vi "Open.vi"(8 "error in (no error)":errorcluster, 11 "Ini-File in":refnum<class "Ini-File.lvclass">) -> (0 "error out":errorcluster, 3 "Ini-File out":refnum<class "Ini-File.lvclass">)   [LabVIEW 2016, in "Configuration.lvlib" / "Ini-File.lvclass"]
doc: "Open connection to ini-file."
uses:
  Ini-File.lvclass
  Ini-File.lvclass/Ini-File.ctl
  <vilib>/Utility/config.llb/NI_LVConfig.lvlib
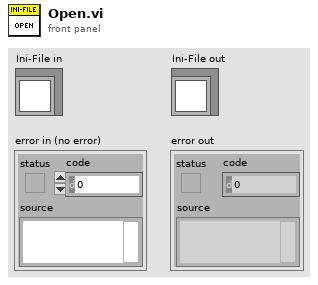
[diagram p1: front panel]
types:
  T1 = typedef "NI_LVConfig.lvlib/Config Data RefNum.ctl" = refnum<k1>
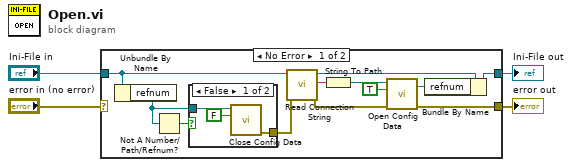
[diagram p0: block diagram]
diagram:
  n1 = case shown="No Error" "error in (no error)" {
    selector: "error in (no error)" -> [_ w21]
    tunnel: [w7 w21] -> w3
    tunnel: [w8 w20] -> w1
    tunnel: "Ini-File in" -> [w11 w20]
    frame No Error {
      n2 = Unbundle By Name(w11) -> ("refnum"=w12:T1)
      n3 = Not A Number/Path/Refnum?(number/path/refnum=w12) -> (NaN/Path/Refnum?=w13:bool)
      n4 = case shown="False" w13 {
        tunnel: [w18 _] -> w14
        tunnel: w12 -> [w17 _]
        frame False {
          n5 = call <vilib>:"Close Config Data.vi"("write file if changed (T)"=FALSE, "refnum"=w17) -> ("error out"=w18:errorcluster)  [unwired: 8 in, 1 out]
        }
        frame True {
        }
      }
      n6 = call-dynamic "Read Connection String.vi"("error in (no error)"=w14, "Interface in"=w11) -> ("error out"=w15:errorcluster, "Connection String"=w6:string, "Interface out"=w10:refnum<class "Ini-File.lvclass">)  [unwired: 7 in]
      n7 = String To Path(string=w6) -> (path=w5:path)
      n8 = call <vilib>:"Open Config Data.vi"("error in (no error)"=w15, "create file if necessary (T)"=TRUE, "configuration file path"=w5) -> ("error out"=w7:errorcluster, "refnum"=w9:T1)  [unwired: 6 in, 1 out]
      n9 = Bundle By Name(cluster=w10, "refnum"=w9) -> (w8:refnum<class "Ini-File.lvclass">)
    }
    frame Error {
    }
  }
  "error out" <- w3
  "Ini-File out" <- w1
